vi "nominal handle list get.vi"(8 "error in (no error)":errorcluster, 9 "out_handle":i32, 10 "index":i32, 11 "list":i32) -> (0 "error out":errorcluster, 1 "out_handle out":i32, 3 "function return":i32)   [LabVIEW 2020, in "client.lvlib"]
doc: "int32_t nominal_handle_list_get(int32_t list, int32_t index, int32_t *out_handle);"
uses:
  client.lvlib
  nominalClient_64.dll
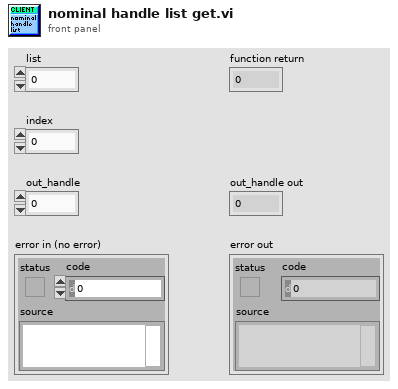
[diagram p1: front panel]
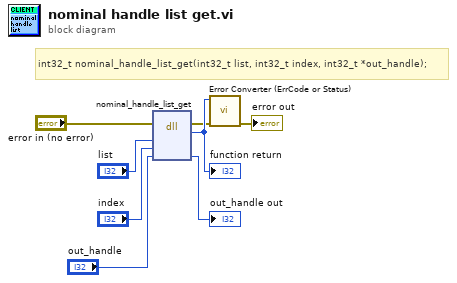
[diagram p0: block diagram]
diagram:
  # "int32_t nominal_handle_list_get(int32_t list, int32_t index, int32_t *out_handle);"
  n1 = dll-call lib="C:/code/labview-client-rs/lv_src/client/nominalClient_64.*" fn="nominal_handle_list_get"(error in="error in (no error)", "list"="list", "index"="index", "out_handle"="out_handle") -> (error out=w2:errorcluster, w8:i32, "out_handle"=→"out_handle out":i32)  [unwired: 4 in, 1 out]
  "function return" <- w8
  n2 = call "Error Converter (ErrCode or Status).vi"("error in (no error)"=w2, "error code"=w8) -> ("error out"=→"error out":errorcluster)  [unwired: 9 in]
